vi "My Acquire Analyze Present.vi"() -> ()   [LabVIEW 2020]
panel:
  out "x-y":dbl
  out "Waveform Graph":dynamicdata(graph)
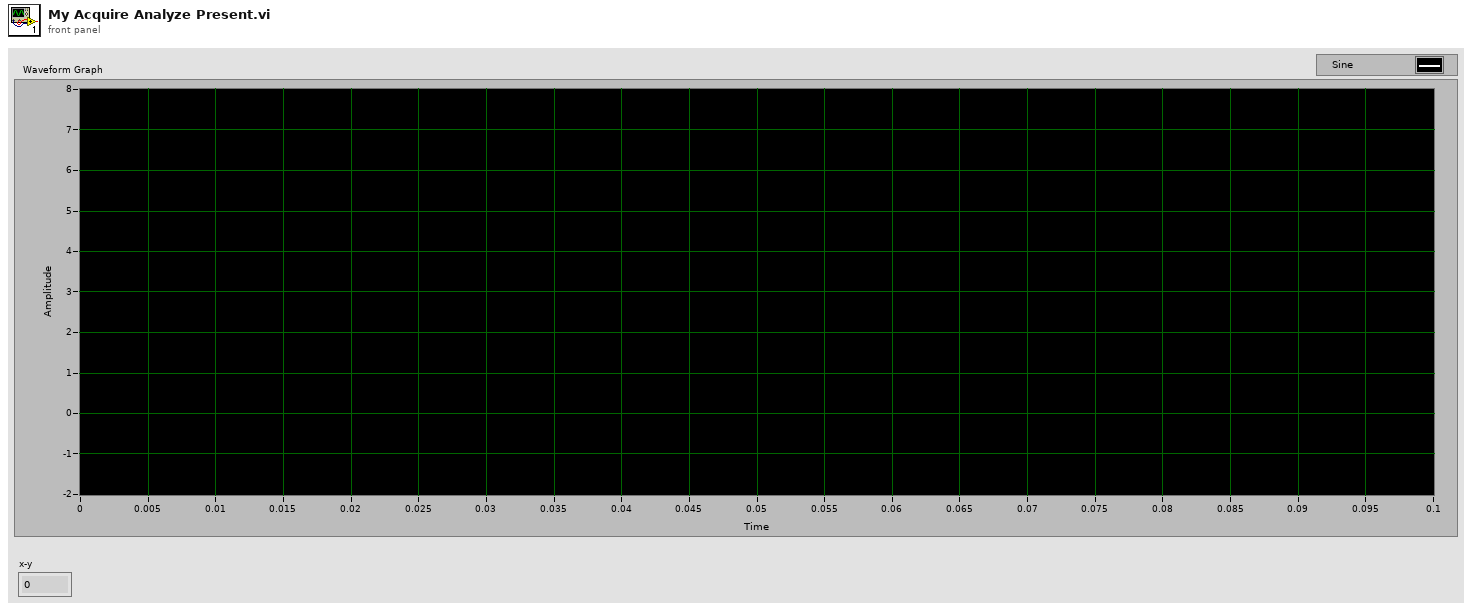
[diagram p1: front panel]
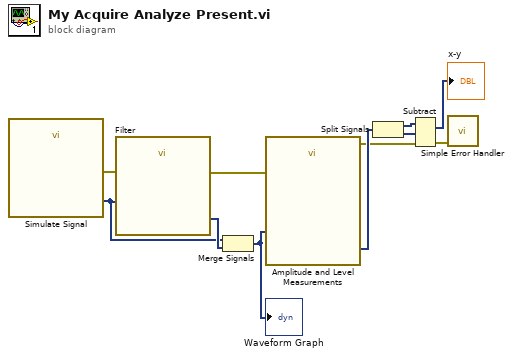
[diagram p0: block diagram]
diagram:
  n1 = call "Simulate Signal"() -> ("Sine"=w7:dynamicdata, "error out"=w9:errorcluster)  [unwired: 14 in]
  n2 = call "Filter"("error in (no error)"=w9, "Signal"=w7) -> ("error out"=w2:errorcluster, "Filtered Signal"=w10:dynamicdata)  [unwired: 8 in]
  n3 = Merge Signals(w7, w10) -> (w6:dynamicdata)
  "Waveform Graph" <- w6
  n4 = call "Amplitude and Level Measurements"("Signals"=w6, "error in (no error)"=w2) -> ("Peak to Peak"=w5:dynamicdata, "error out"=w1:errorcluster)  [unwired: 12 in]
  n5 = Split Signals(w5) -> (w4:dynamicdata, w3:dynamicdata)  [unwired: 2 in]
  n6 = Subtract(1:w3, 2:w4, 4:w1) -> (0:→"x-y":dynamicdata, 3:w8:errorcluster)
  n7 = call <vilib>:"Simple Error Handler.vi"("error in (no error)"=w8) -> ()  [unwired: 4 in, 5 out]
